vi "Test TCRS Update Setpoint.vi"(8 "error in (no error)":errorcluster, 11 "Thermal Chamber Response Simlator Test In":refnum<class "Thermal Chamber Response Simlator Test.lvclass">) -> (0 "error out":errorcluster, 3 "Thermal Chamber Response Simlator Test Out":refnum<class "Thermal Chamber Response Simlator Test.lvclass">)   [LabVIEW 2020, in "Thermal Chamber Response Simlator Test.lvclass"]
uses:
  Thermal Chamber Response Simlator Test.lvclass
  C:/Program Files (x86)/National Instruments/LabVIEW 2020/vi.lib/Astemes/LUnit/Test Case.lvclass
  Thermal Chamber Response Simlator/Thermal Chamber Response Simlator.lvclass
  Thermal Chamber Response Simlator/Thermal Chamber Response Simlator.lvclass/Thermal Chamber Response Simlator.ctl
  <vilib>/Astemes/LUnit/Test Case.lvclass/Test Case.ctl
  <vilib>/Astemes/LUnit/Palette/Pass If Equal.vi/cbf50e99-f124-4847-863a-8e9794d3dede.vi
  <vilib>/Astemes/LUnit/Palette/Pass.vi
  <vilib>/Astemes/LUnit/Palette/Fail.vi
  <vilib>/Astemes/LUnit/Compare Variants.vi
  <vilib>/Astemes/LUnit/Describe Comparison.vi
  <vilib>/Astemes/LUnit/Set Assertion Type.vi
  <vilib>/Astemes/LUnit/Add test result.vi
  <vilib>/Astemes/LUnit/Variant to string.vi
  <vilib>/Astemes/LUnit/LUnit Record Assertion Result.vi
  <vilib>/Astemes/LUnit/LUnit Aggregate Assertion Results.vi
  <vilib>/Astemes/LUnit/Method Result/LUnit Merge Status.vi
  <vilib>/Astemes/LUnit/LUnit Concatenate result strings.vi
  Thermal Chamber Response Simlator/Private/Get Current Time if Not Set.vi
  <vilib>/Utility/Data Type/Get Type Information.vi
  <vilib>/Utility/LVClass/Get LV Class Name.vi
  <vilib>/Astemes/LUnit/Test Case.lvclass
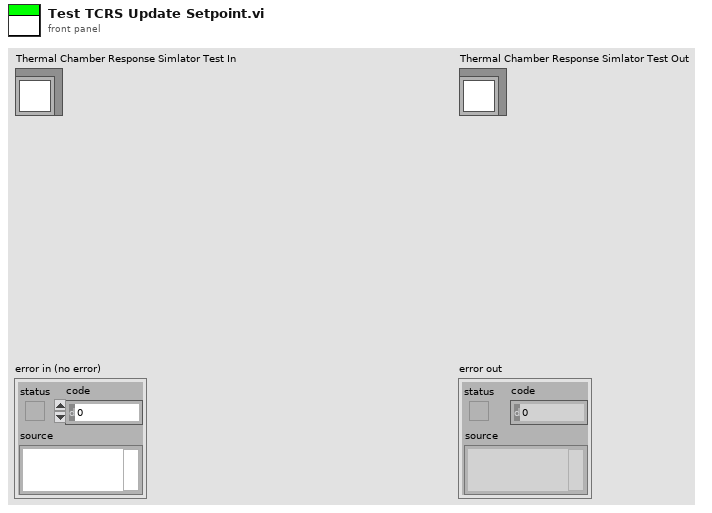
[diagram p1: front panel]
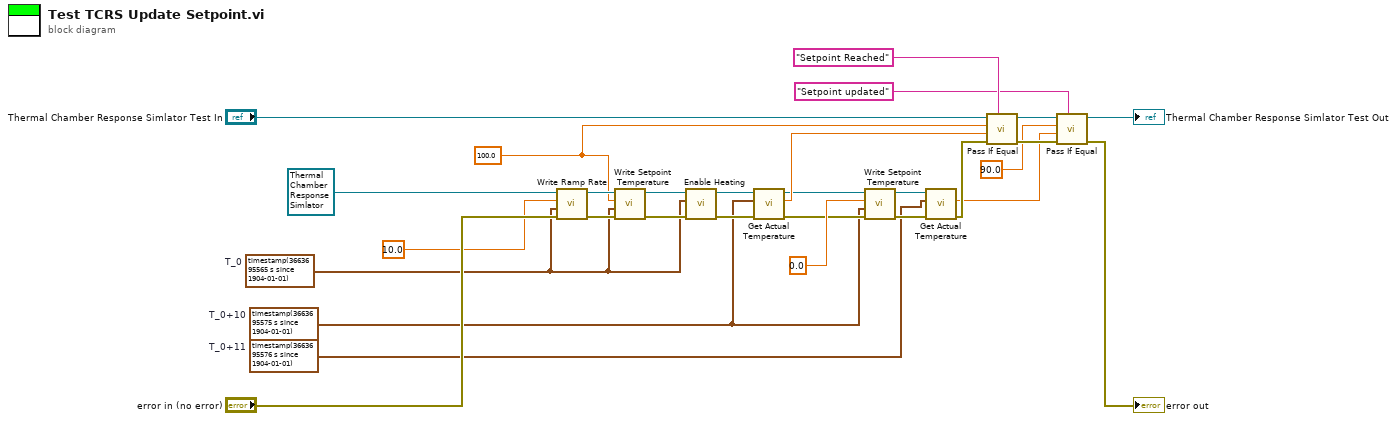
[diagram p0: block diagram]
diagram:
  w5 = timestamp(3663695576 s since 1904-01-01)  # T_0+11
  w16 = 100.0 ("Setpoint Temperature [degC]")
  w2 = timestamp(3663695575 s since 1904-01-01)  # T_0+10
  w1 = timestamp(3663695565 s since 1904-01-01)  # T_0
  n1 = call "Write Ramp Rate.vi"("error in (no error)"="error in (no error)", "Time Stamp"=w1, "Ramp Rate [degC/s]"=10.0, "Thermal Chamber Response Simlator In"=refnum<class "Thermal Chamber Response Simlator.lvclass"> refnum ("Thermal Chamber Response Simlator.lvclass")) -> ("error out"=w25:errorcluster, "Thermal Chamber Response Simlator Out"=w23:refnum<class "Thermal Chamber Response Simlator.lvclass">)  [unwired: 6 in]
  n2 = call "Write Setpoint Temperature.vi"("error in (no error)"=w25, "Update Time"=w1, "Setpoint Temperature [degC]"=w16, "Thermal Chamber Response Simlator In"=w23) -> ("error out"=w24:errorcluster, "Thermal Chamber Response Simlator Out"=w22:refnum<class "Thermal Chamber Response Simlator.lvclass">)  [unwired: 6 in]
  n3 = call "Enable Heating.vi"("error in (no error)"=w24, "Start Time"=w1, "Thermal Chamber Response Simlator In"=w22) -> ("error out"=w20:errorcluster, "Thermal Chamber Response Simlator Out"=w19:refnum<class "Thermal Chamber Response Simlator.lvclass">)  [unwired: 7 in]
  n4 = call "Get Actual Temperature.vi"("error in (no error)"=w20, "Time Stamp"=w2, "Thermal Chamber Response Simlator In"=w19) -> ("error out"=w12:errorcluster, "Actual Temperature [degC]"=w17:dbl, "Thermal Chamber Response Simlator Out"=w15:refnum<class "Thermal Chamber Response Simlator.lvclass">)  [unwired: 6 in]
  n5 = call "Write Setpoint Temperature.vi"("error in (no error)"=w12, "Update Time"=w2, "Setpoint Temperature [degC]"=0.0, "Thermal Chamber Response Simlator In"=w15) -> ("error out"=w13:errorcluster, "Thermal Chamber Response Simlator Out"=w14:refnum<class "Thermal Chamber Response Simlator.lvclass">)  [unwired: 6 in]
  n6 = call "Get Actual Temperature.vi"("error in (no error)"=w13, "Time Stamp"=w5, "Thermal Chamber Response Simlator In"=w14) -> ("error out"=w11:errorcluster, "Actual Temperature [degC]"=w3:dbl)  [unwired: 6 in, 1 out]
  n7 = call <vilib>:"Pass If Equal.vi"("Description"="Setpoint Reached", "error in (no error)"=w11, "Actual"=w17, "Expected"=w16, "LUnit Test Case In"="Thermal Chamber Response Simlator Test In") -> ("error out"=w10:errorcluster, "LUnit Test Case Out"=w7:refnum<class "Thermal Chamber Response Simlator Test.lvclass">)  [unwired: 5 in]
  n8 = call <vilib>:"Pass If Equal.vi"("Description"="Setpoint updated", "error in (no error)"=w10, "Actual"=w3, "Expected"=90.0 ("Setpoint Temperature [degC]"), "LUnit Test Case In"=w7) -> ("error out"=→"error out":errorcluster, "LUnit Test Case Out"=→"Thermal Chamber Response Simlator Test Out":refnum<class "Thermal Chamber Response Simlator Test.lvclass">)  [unwired: 5 in]
